vi "set_single_outlet.vi"(9 "Switch state":bool, 10 "Outlet #":i32, 11 "IP / Hostname":string="172.20.125.112") -> ()   [LabVIEW 2021]
panel:
  out "return":string="1\r\n"
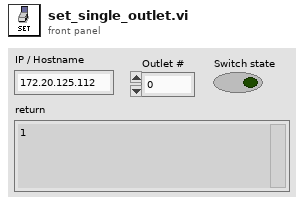
[diagram p1: front panel]
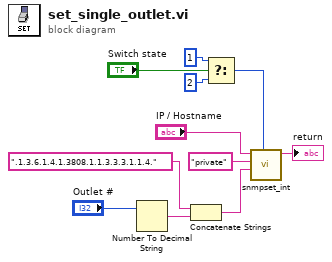
[diagram p0: block diagram]
diagram:
  n1 = Number To Decimal String(number="Outlet #") -> (decimal integer string=w8:string)  [unwired: 1 in]
  n2 = Concatenate Strings(".1.3.6.1.4.1.3808.1.1.3.3.3.1.1.4." ("OID"), w8) -> (w7:string)
  n3 = Select(t=1, s="Switch state", f=2) -> (s? t:f=w4:i32)
  n4 = call "snmpset_int.vi"("value"=w4, "OID"=w7, "community"="private", "IP / Hostname"="IP / Hostname") -> ("return"=→"return":string)  [unwired: 6 in, 1 out]
